vi "shift_append_to_end.vi"(9 "new element":dbl, 10 "input array":dbl[](array[numeric])) -> (2 "output array":dbl[](array[numeric]))   [LabVIEW 2010]
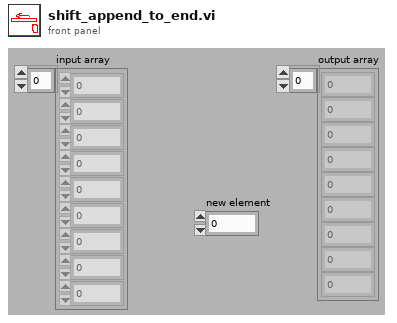
[diagram p1: front panel]
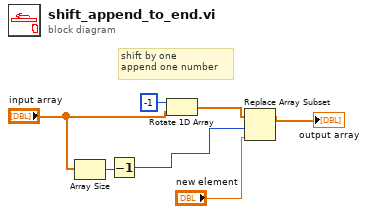
[diagram p0: block diagram]
diagram:
  # "shift by one \nappend one number"
  n1 = Array Size(array="input array") -> (size(s)=w2:i32)
  n2 = Decrement(x=w2) -> (x-1=w1:i32)
  n3 = Rotate 1D Array(1:"input array", 2:-1 ("n")) -> (0:w7:dbl[])
  n4 = Replace Array Subset(array=w7, new element="new element", index=w1) -> (→"output array":dbl[])
